vi "Recipe.vi"(8 "error in (no error)":errorcluster, 10 "Notifiers":T1, 11 "All Message Queue Cluster":T2) -> (0 "error out":errorcluster)   [LabVIEW 2013]
uses:
  Lib Log/Logging.lvlib
  Lib QMH/MessageQueues.lvlib
  Lib QMH/Message Cluster.ctl
  Lib QMH/AllMessageQueue Cluster.ctl
  Lib Notifier/Notifier.ctl
  Lib Notifier/Notifier.lvlib
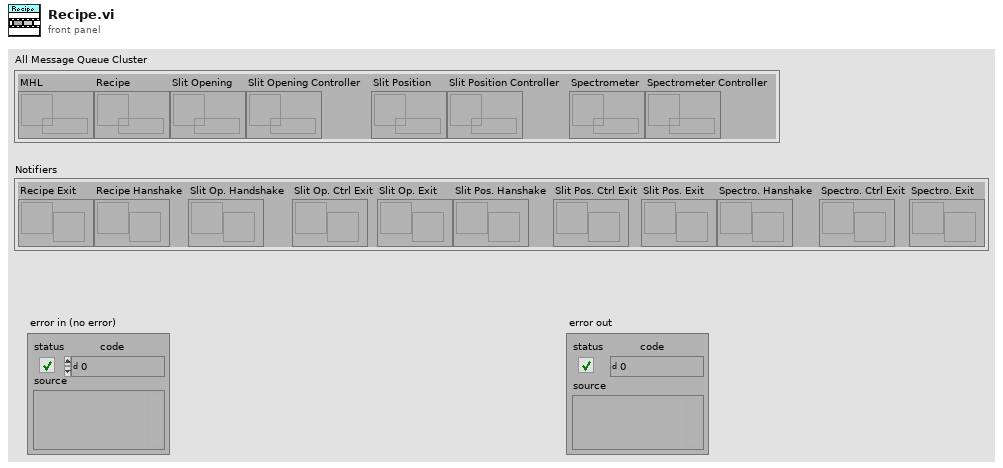
[diagram p1: front panel]
types:
  T1 = typedef "Notifier.lvlib/Notifier.ctl" = cluster{"Recipe Exit":refnum<notifier>, "Recipe Hanshake":refnum<notifier>, "Slit Op. Handshake":refnum<notifier>, "Slit Op. Ctrl Exit":refnum<notifier>, "Slit Op. Exit":refnum<notifier>, "Slit Pos. Hanshake":refnum<notifier>, "Slit Pos. Ctrl Exit":refnum<notifier>, "Slit Pos. Exit":refnum<notifier>, "Spectro. Hanshake":refnum<notifier>, "Spectro. Ctrl Exit":refnum<notifier>, "Spectro. Exit":refnum<notifier>}
  T2 = typedef "MessageQueues.lvlib/AllMessageQueue Cluster.ctl" = cluster{"MHL":refnum<queue>, "Recipe":refnum<queue>, "Slit Opening":refnum<queue>, "Slit Opening Controller":refnum<queue>, "Slit Position":refnum<queue>, "Slit Position Controller":refnum<queue>, "Spectrometer":refnum<queue>, "Spectrometer Controller":refnum<queue>}
  T3 = enum16{"open", "replace", "create", "open or create", "replace or create", "replace or create with confirmation"}
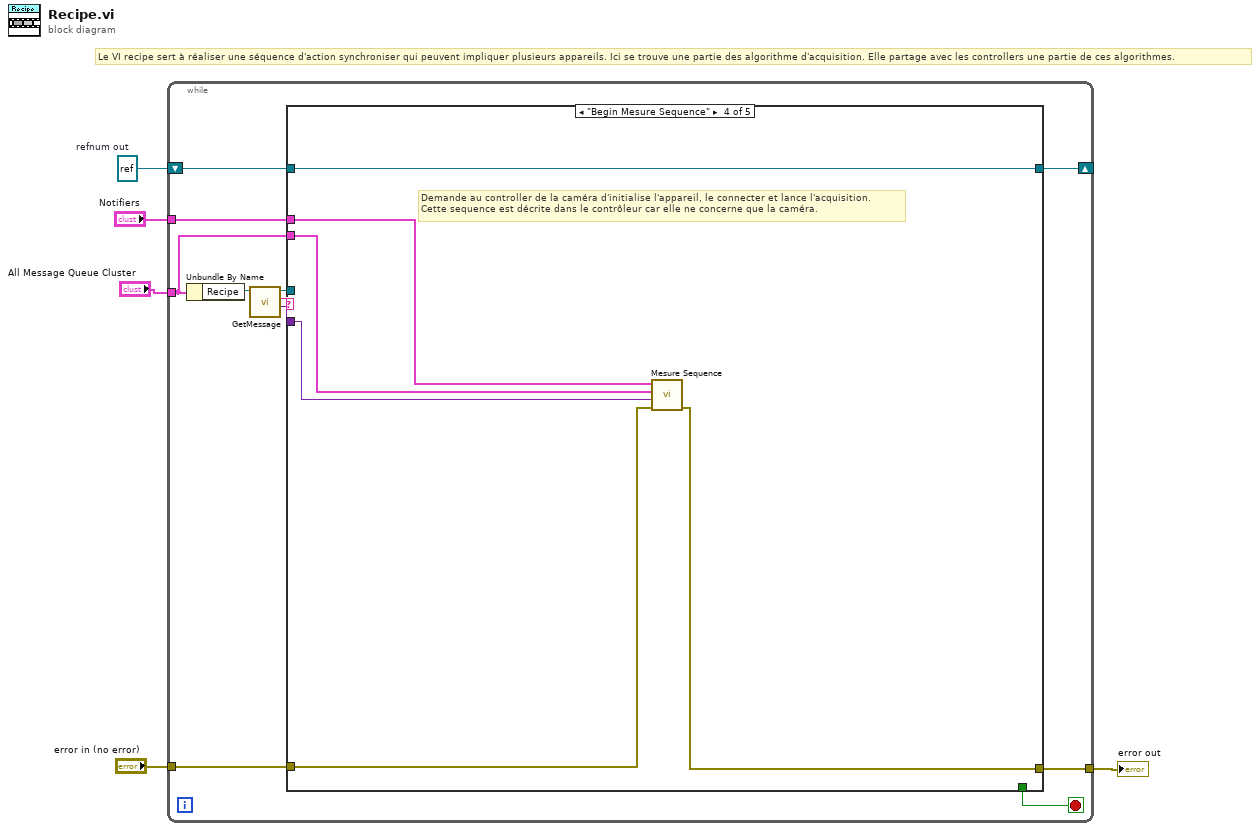
[diagram p0: block diagram]
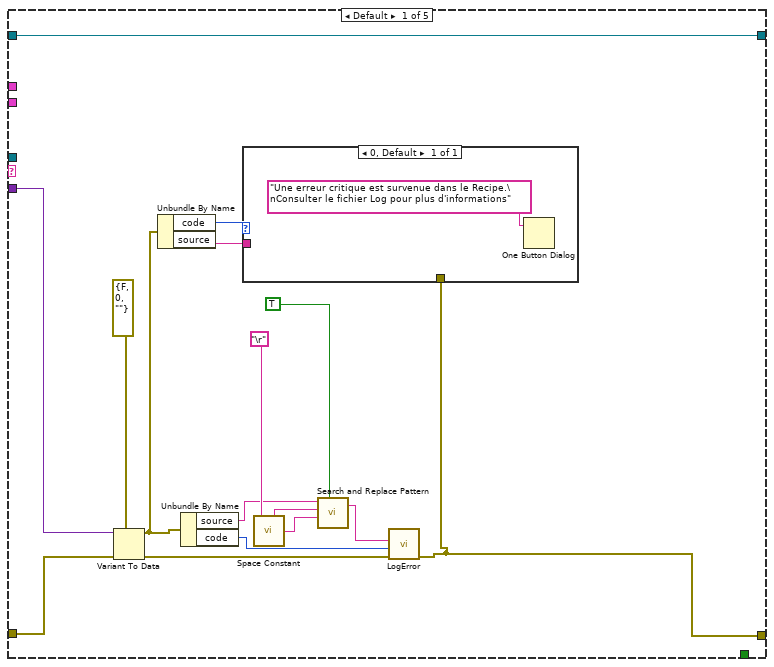
[diagram p2: hidden frame]
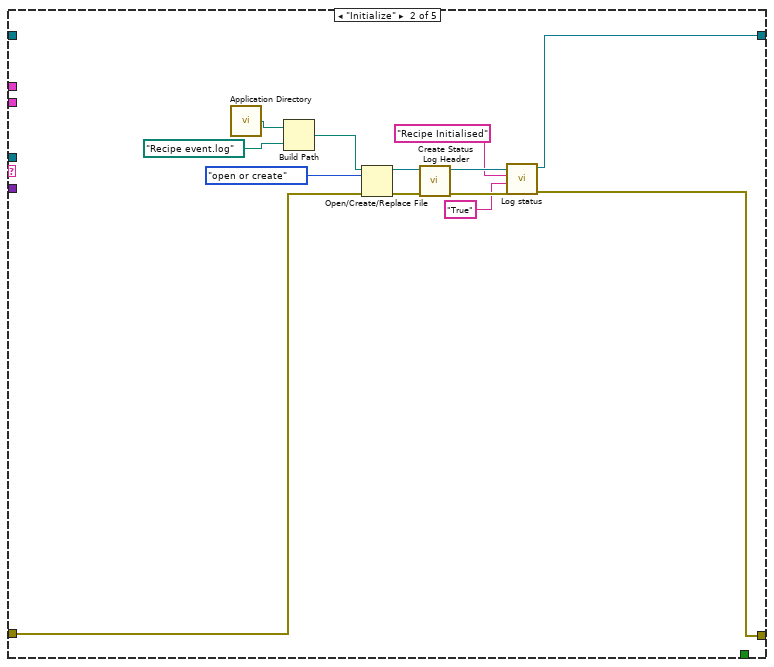
[diagram p3: hidden frame]
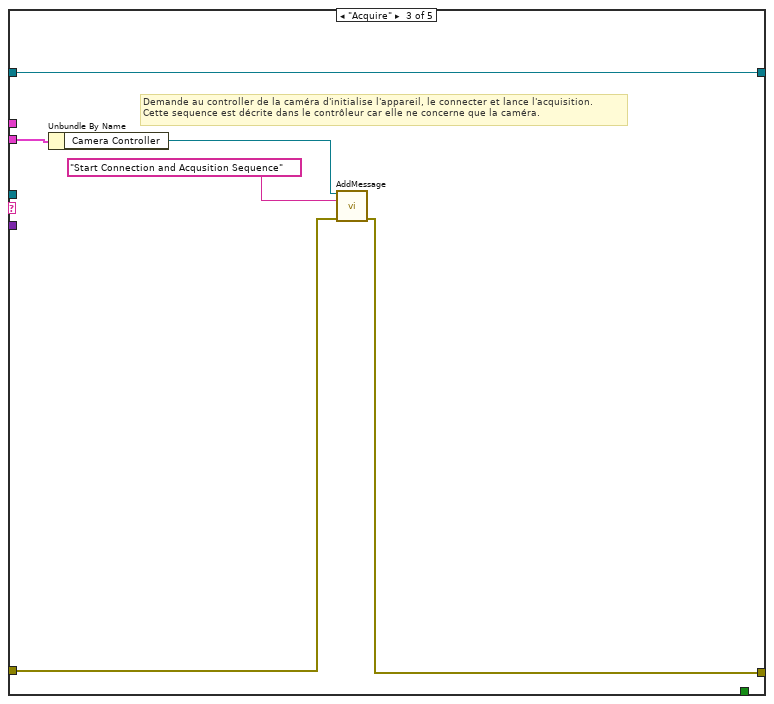
[diagram p4: hidden frame]
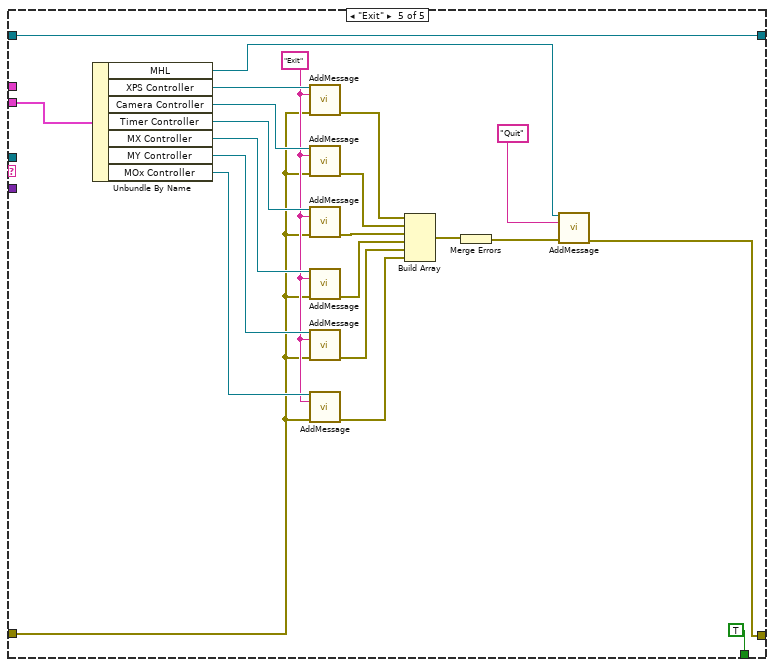
[diagram p5: hidden frame]
diagram:
  w2 = refnum<file> refnum  # refnum out
  # "Le VI recipe sert à réaliser une séquence d'action synchroniser qui peuvent impliquer plusieurs appareils. Ici se trouve une partie des algorithme d'acquisition. Elle partage avec les controllers une partie de ces algorithmes."
  n1 = while {
    tunnel: "All Message Queue Cluster" -> [w14]
    tunnel: "Notifiers" -> [w15]
    tunnel: "error in (no error)" -> [w13]
    tunnel: [w6] -> w1
    shift-right: [w8] -> _
    shift-left: w2 -> [w7]
    stop <- w12 stop-if-true
    n2 = Unbundle By Name(w14) -> ("Recipe"=w16:refnum<queue>)
    n3 = call "GetMessage.vi"("Message queue"=w16) -> ("Data"=w9:variant, "Message"=w10:string, "Dup Message Queue"=w11:refnum<queue>)  [unwired: 7 in, 1 out]
    n4 = case shown="\"Begin Mesure Sequence\"" w10 {
      tunnel: w15 -> [_ _ _ w52 _]
      tunnel: w14 -> [_ _ w50 w53 w77]
      tunnel: w13 -> [w19 w41 w48 w56 w69]
      tunnel: [_ _ _ _ TRUE] -> w12
      tunnel: w11 -> [_ _ _ _ _]
      tunnel: w9 -> [w17 _ _ w54 _]
      tunnel: [w31 w33 w51 w57 w79] -> w8
      tunnel: w7 -> [w31 _ w51 w57 w79]
      tunnel: [w18 w37 w47 w55 w60] -> w6
      frame Default {
        n5 = Variant To Data(error in=w19, type=errorcluster {"status"=FALSE, "code"=0, "source"=""} ("error in (no error)"), Variant=w17) -> (data=w30:errorcluster, error out=w21:errorcluster)
        n6 = Unbundle By Name(w30) -> ("code"=w28:i32, "source"=w29:string)
        n7 = Unbundle By Name(w30) -> ("source"=w23:string, "code"=w22:i32)
        n8 = call <vilib>:"Space Constant.vi"() -> ("String"=w25:string)
        n9 = call <vilib>:"Search and Replace Pattern.vi"("string"=w23, "regular expression (\"\")"="\r", "replace string (\"\")"=w25, "replace all? (F)"=TRUE) -> ("result string"=w26:string)  [unwired: 1 in, 1 out]
        n10 = call "LogError.vi"("entrée d'erreur"=w21, "Code"=w22, "Source"=w26) -> ("error out"=w18:errorcluster)  [unwired: 7 in, 1 out]
        n11 = case shown="0, Default" w28 {
          tunnel: w29 -> [_]
          tunnel: w18 -> [_]
          frame 0, Default {
            n12 = One Button Dialog(message="Une erreur critique est survenue dans le Recipe.\nConsulter le fichier Log pour plus d'informations" ("chaîne de format")) -> ()  [unwired: 1 in, 1 out]
          }
        }
      }
      frame "Initialize" {
        n13 = call <vilib>:"Application Directory.vi"() -> ("Application Directory"=w42:path)
        n14 = Build Path(base path=w42, name or relative path=path "Recipe event.log") -> (appended path=w44:path)
        n15 = Open/Create/Replace File(file path (use dialog)=w44, error in=w41, operation (0:open)=T3."open or create" ("opération (0 : open)")) -> (refnum out=w39:refnum<file>, error out=w40:errorcluster)  [unwired: 3 in, 1 out]
        n16 = call "Create Status Log Header.vi"("entrée d'erreur"=w40, "Log File Refnum In"=w39) -> ("sortie d'erreur"=w38:errorcluster, "Log File Refnum out"=w36:refnum<file>)  [unwired: 8 in]
        n17 = call "Log status.vi"("entrée d'erreur"=w38, "Event Data String (-)"="True", "Event string"="Recipe Initialised", "Log File Refnum In"=w36) -> ("error out"=w37:errorcluster, "Log File Refnum out"=w33:refnum<file>)  [unwired: 6 in]
      }
      frame "Acquire" {
        # "Demande au controller de la caméra d'initialise l'appareil, le connecter et lance l'acquisition.\nCette sequence est décrite dans le contrôleur car elle ne concerne que la caméra."
        n18 = Unbundle By Name(w50) -> ("Camera Controller"=w46:refnum<queue>)
        n19 = call "AddMessage.vi"("Message queue"=w46, "Message"="Start Connection and Acqusition Sequence", "entrée d'erreur (pas d'erreur)"=w48) -> ("error out"=w47:errorcluster)  [unwired: 11 in, 1 out]
      }
      frame "Begin Mesure Sequence" {
        # "Demande au controller de la caméra d'initialise l'appareil, le connecter et lance l'acquisition.\nCette sequence est décrite dans le contrôleur car elle ne concerne que la caméra."
        n20 = call "Mesure Sequence.vi"("error in"=w56, "Data"=w54, "All Message Queue Cluster"=w53, "Notifiers"=w52) -> ("error out"=w55:errorcluster)  [unwired: 7 in]
      }
      frame "Exit" {
        w70 = "Exit" ("Message")
        n21 = Unbundle By Name(w77) -> ("MHL"=w58:refnum<queue>, "XPS Controller"=w76:refnum<queue>, "Camera Controller"=w75:refnum<queue>, "Timer Controller"=w74:refnum<queue>, "MX Controller"=w73:refnum<queue>, "MY Controller"=w72:refnum<queue>, "MOx Controller"=w71:refnum<queue>)
        n22 = call "AddMessage.vi"("Message queue"=w76, "Message"=w70, "entrée d'erreur (pas d'erreur)"=w69) -> ("error out"=w68:errorcluster)  [unwired: 11 in, 1 out]
        n23 = call "AddMessage.vi"("Message queue"=w75, "Message"=w70, "entrée d'erreur (pas d'erreur)"=w69) -> ("error out"=w67:errorcluster)  [unwired: 11 in, 1 out]
        n24 = call "AddMessage.vi"("Message queue"=w74, "Message"=w70, "entrée d'erreur (pas d'erreur)"=w69) -> ("error out"=w66:errorcluster)  [unwired: 11 in, 1 out]
        n25 = call "AddMessage.vi"("Message queue"=w73, "Message"=w70, "entrée d'erreur (pas d'erreur)"=w69) -> ("error out"=w65:errorcluster)  [unwired: 11 in, 1 out]
        n26 = call "AddMessage.vi"("Message queue"=w72, "Message"=w70, "entrée d'erreur (pas d'erreur)"=w69) -> ("error out"=w64:errorcluster)  [unwired: 11 in, 1 out]
        n27 = call "AddMessage.vi"("Message queue"=w71, "Message"=w70, "entrée d'erreur (pas d'erreur)"=w69) -> ("error out"=w63:errorcluster)  [unwired: 11 in, 1 out]
        n28 = Build Array(w68, w67, w66, w65, w64, w63) -> (w62:errorcluster[])
        n29 = Merge Errors(w62) -> (w61:errorcluster)
        n30 = call "AddMessage.vi"("Message queue"=w58, "Message"="Quit", "entrée d'erreur (pas d'erreur)"=w61) -> ("error out"=w60:errorcluster)  [unwired: 11 in, 1 out]
      }
    }
  }
  "error out" <- w1
